vi "GEA2_Reregister.vi"(5 "Board Index":i32 min=0 max=10 step=1, 7 "Event Registration In":refnum<event-registration>, 11 "Error In":errorcluster) -> (4 "GEA2 Reference Out":refnum<k24>, 6 "Board ID":string, 8 "Event Registration Out":refnum<event-registration>, 15 "Error Out":errorcluster)   [LabVIEW 2016]
uses:
  C:/Automation/DLLs/PC Dot Net/GeaCommunication.dll
  Common/LabVIEW GEA2 Toolkit/LabVIEW_GEA2_Toolkit.lvlibp/type defs/Data Out.ctl
  Common/LabVIEW GEA2 Toolkit/LabVIEW_GEA2_Toolkit.lvlibp/advanced/GEA2 Message Received Event Handler.vi
  Common/LabVIEW GEA2 Toolkit/LabVIEW_GEA2_Toolkit.lvlibp
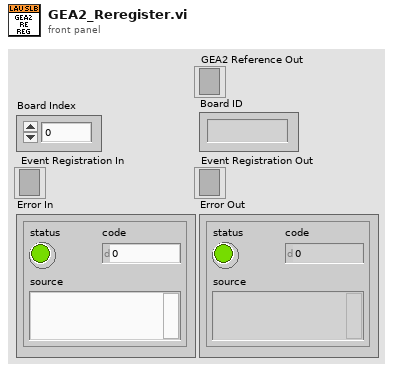
[diagram p1: front panel]
types:
  T1 = typedef "LabVIEW_GEA2_Toolkit.lvlibp/Data Out.ctl" = cluster{"Source":u8, "Destination":u8, "Command":u8, "Length":u8, "CRC":u16, "Message":string}
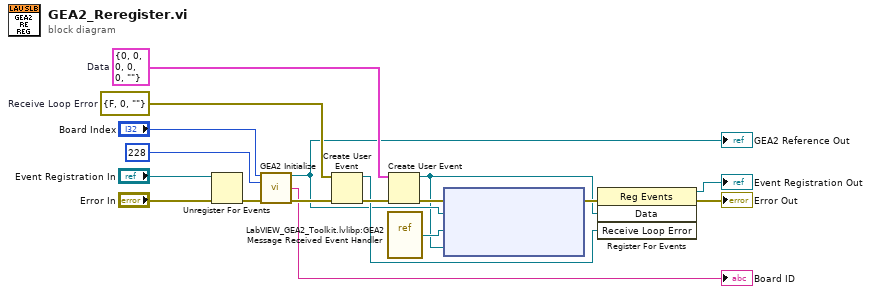
[diagram p0: block diagram]
diagram:
  w15 = errorcluster {"status"=FALSE, "code"=0, "source"=""}  # Receive Loop Error
  w16 = T1 {"Source"=0, "Destination"=0, "Command"=0, "Length"=0, "CRC"=0, "Message"=""}  # Data
  n1 = Unregister For Events(event registration refnum="Event Registration In", error in="Error In") -> (error out=w9:errorcluster)
  n2 = call "GEA2 Initialize.vi"("Board Index"="Board Index", "Source Address"=u8 228, "error in"=w9) -> ("GEA2 Reference Out"=w8:refnum<k24>, "Board ID"=→"Board ID":string, "error out"=w10:errorcluster)  [unwired: 10 in]
  "GEA2 Reference Out" <- w8
  n3 = Create User Event(user event datatype=w15, error in=w10) -> (user event=w13:refnum<user-event>, error out=w14:errorcluster)
  n4 = vi-ref "LabVIEW_GEA2_Toolkit.lvlibp:GEA2 Message Received Event Handler.vi"() -> (w6:refnum<vi>)
  n5 = Create User Event(user event datatype=w16, error in=w14) -> (user event=w4:refnum<user-event>, error out=w11:errorcluster)
  n6 = node(w11, w8, w6, w4) -> (w12:errorcluster)  [unwired: 1 in, 1 out]
  n7 = register-events(error in=w12, w4, w13) -> (reference out=→"Event Registration Out":refnum<event-registration>, error out=→"Error Out":errorcluster)  [unwired: 1 in]
